vi "Create Contour.vi"(7 "3D Contour Property":T5={"General Property"={"Plot Name"="", "Coordinate System"=enum."Cartesian", "Opacity"=0.0}, "Projection Property"={"Draw XY"=FALSE, "Draw YZ"=FALSE, "Draw XZ"=FALSE}, "Plot Property"={"Line Style"=enum."None", "Line Width"=2.0, "Line Color"=0, "Antialiasing"=FALSE, "Color Ramp Cluster"={"Color Ramp Style"=enum."None", "Color Ramp Array"=[16711934, 393471, 57855, 4390754, 16449346, 16744722, 16711680], "Color Ramp Index"=[45, 91, 133, 175, 219, 255], "Interpolate?"=FALSE, "Logarithm?"=FALSE}}, "Contour Property"={"Contour Type"=enum."Contour", "Axis Basis"=enum."Z-Axis", "Level List"=[], "Level Mode"=enum."Levels", "Levels"=0, "Interval"=0.0}}, 8 "error in (no error)":errorcluster, 9 "Actual Transform In":T1, 10 "Plot Representation In":T3, 11 "Plot Object In":refnum<vi>) -> (0 "error out":errorcluster, 1 "Actual Transform Out":T1, 2 "Plot Representation Out":T3, 3 "Plot Object Out":refnum<vi>, 4 "Contour Object Out":refnum<vi>)   [LabVIEW 2020, in "3D Contour.lvclass"]
uses:
  <vilib>/Math Plots/3D Math Plots/3D Contour/3D Contour/3D Contour.lvclass
  <vilib>/Math Plots/3D Math Plots/3D Contour/3D Contour/Typedef/3D Contour Property.ctl
  <vilib>/Math Plots/3D Math Plots/3D Plot/3D Plot/Typedef/Line Type.ctl
  <vilib>/Math Plots/3D Math Plots/3D Plot/3D Plot/Typedef/Color Ramp Cluster.ctl
  <vilib>/Math Plots/3D Math Plots/3D Plot/3D Plot/Typedef/Plot Representation.ctl
  <vilib>/Math Plots/3D Math Plots/3D Plot/3D Plot/Typedef/Range Clusters.ctl
  <vilib>/Math Plots/3D Math Plots/3D Plot/3D Plot/Typedef/Mesh Data.ctl
  <vilib>/Math Plots/3D Math Plots/3D Plot/3D Plot/Typedef/Actual Transform.ctl
  <vilib>/picture/3D Picture Control/NI_3D Picture Control.lvlib
  <vilib>/Math Plots/3D Math Plots/3D Plot/3D Plot/3D Plot.lvclass
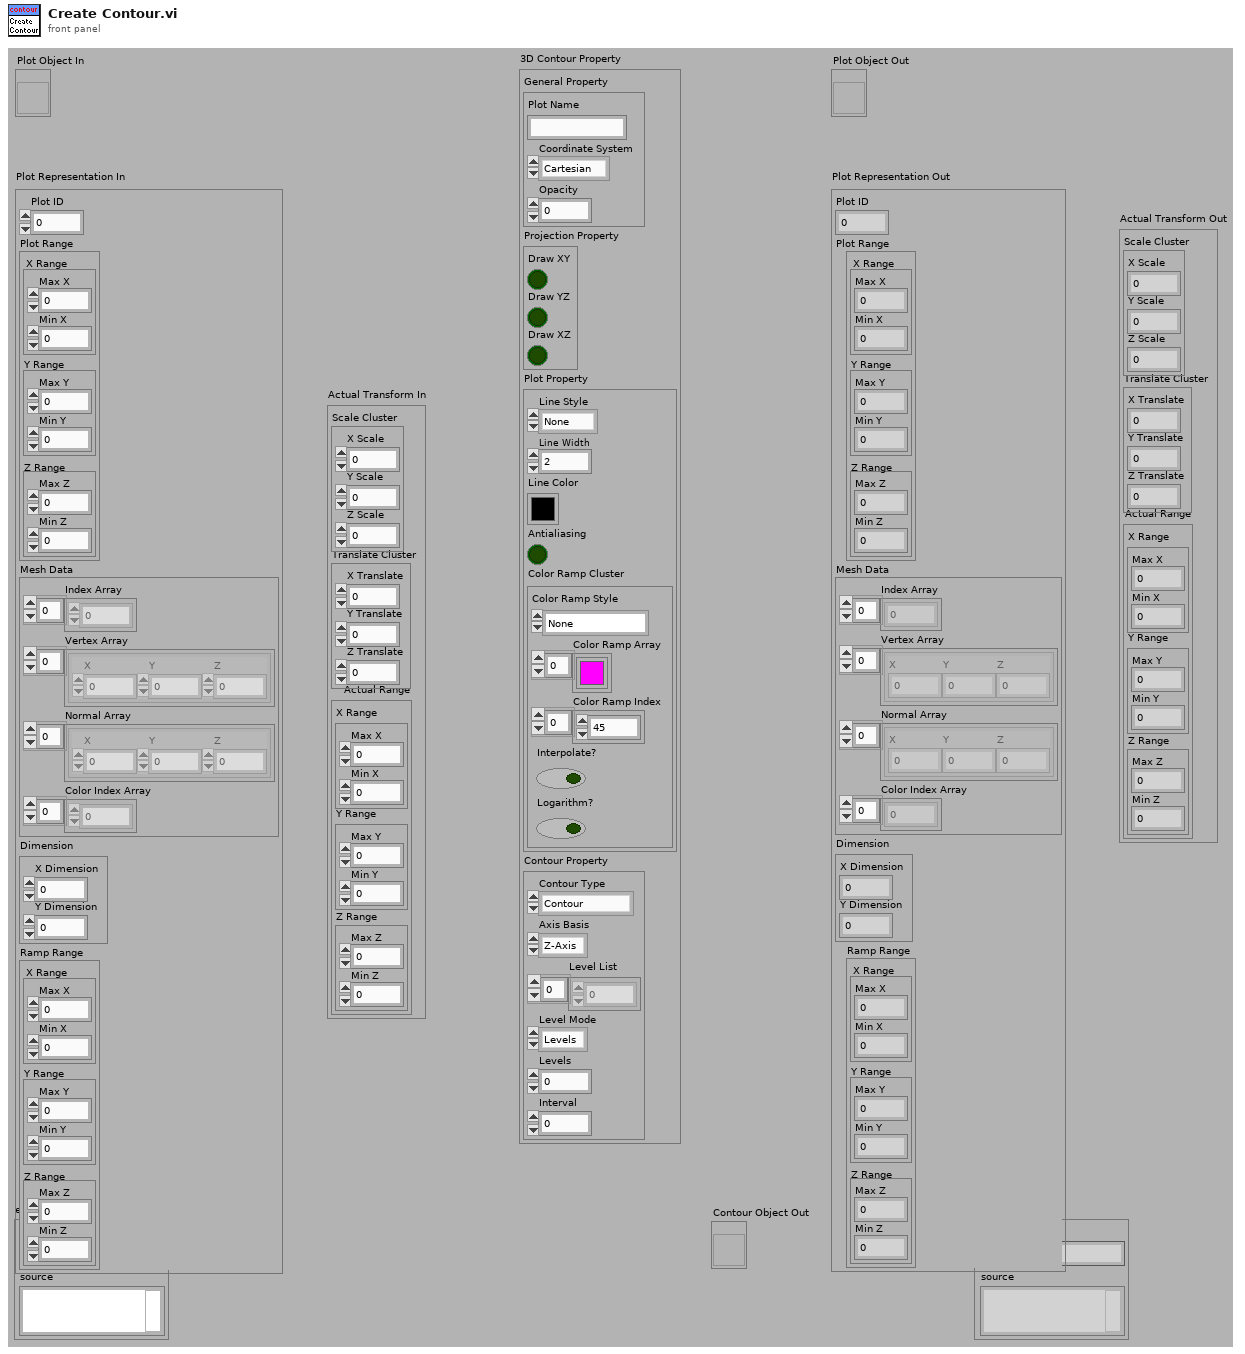
[diagram p1: front panel]
types:
  T1 = typedef "3D Plot.lvclass/Actual Transform.ctl" = cluster{"Scale Cluster":cluster{"X Scale":sgl, "Y Scale":sgl, "Z Scale":sgl}, "Translate Cluster":cluster{"X Translate":sgl, "Y Translate":sgl, "Z Translate":sgl}, "Actual Range":T2}
  T2 = typedef "3D Plot.lvclass/Range Clusters.ctl" = cluster{"X Range":cluster{"Max X":sgl, "Min X":sgl}, "Y Range":cluster{"Max Y":sgl, "Min Y":sgl}, "Z Range":cluster{"Max Z":sgl, "Min Z":sgl}}
  T3 = typedef "3D Plot.lvclass/Plot Representation.ctl" = cluster{"Plot ID":i32, "Plot Range":T2, "Mesh Data":T4, "Dimension":cluster{"X Dimension":i32, "Y Dimension":i32}, "Ramp Range":T2}
  T4 = typedef "3D Plot.lvclass/Mesh Data.ctl" = cluster{"Index Array":u32[], "Vertex Array":cluster{"X":sgl, "Y":sgl, "Z":sgl}[], "Normal Array":cluster{"X":sgl, "Y":sgl, "Z":sgl}[], "Color Index Array":i32[]}
  T5 = typedef "3D Contour.lvclass/3D Contour Property.ctl" = cluster{"General Property":cluster{"Plot Name":string, "Coordinate System":enum16{"Cartesian", "Cylindrical", "Spherical"}, "Opacity":sgl}, "Projection Property":cluster{"Draw XY":bool, "Draw YZ":bool, "Draw XZ":bool}, "Plot Property":cluster{"Line Style":T6, "Line Width":sgl, "Line Color":u32, "Antialiasing":bool, "Color Ramp Cluster":T7}, "Contour Property":cluster{"Contour Type":enum16{"Contour", "Contour with surface"}, "Axis Basis":enum16{"X-Axis", "Y-Axis", "Z-Axis"}, "Level List":sgl[], "Level Mode":enum16{"Levels", "Interval", "Level List"}, "Levels":u16, "Interval":sgl}}
  T6 = typedef "3D Plot.lvclass/Line Type.ctl" = enum16{"None", "Solid", "Dash", "Dot", "Dash Dot"}
  T7 = typedef "3D Plot.lvclass/Color Ramp Cluster.ctl" = cluster{"Color Ramp Style":enum16{"None", "Shaded", "Color spectrum", "Grey scale", "Custom"}, "Color Ramp Array":u32[], "Color Ramp Index":i32[], "Interpolate?":bool, "Logarithm?":bool}
  T8 = enum16{"Points", "Lines", "Line Strip", "Line Loop", "Triangles", "Triangle Strip", "Triangle Fan", "Quads", "Quad Strip", "Polygon"}
  T9 = cluster{"Contour Type":enum16{"Contour", "Contour with surface"}, "Axis Basis":enum16{"X-Axis", "Y-Axis", "Z-Axis"}, "Level List":sgl[], "Level Mode":enum16{"Levels", "Interval", "Level List"}, "Levels":u16, "Interval":sgl}
  T10 = enum16{"Overall", "Per Primitive", "Per Vertex", "Binding Off"}
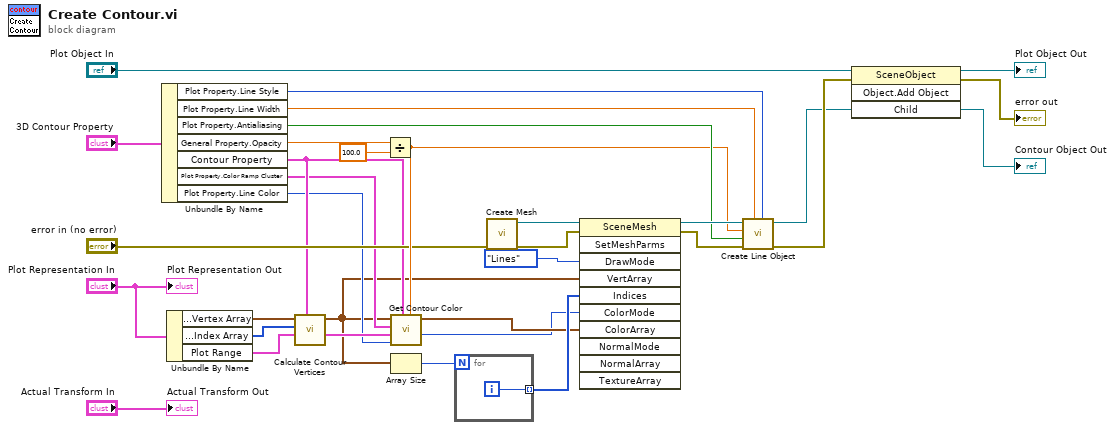
[diagram p0: block diagram]
diagram:
  n1 = Unbundle By Name("3D Contour Property") -> ("Plot Property.Line Style"=w13:T6, "Plot Property.Line Width"=w14:sgl, "Plot Property.Antialiasing"=w12:bool, "General Property.Opacity"=w20:sgl, "Contour Property"=w4:T9, "Plot Property.Color Ramp Cluster"=w3:T7, "Plot Property.Line Color"=w2:u32)
  n2 = Unbundle By Name("Plot Representation In") -> ("Mesh Data.Vertex Array"=w8:cluster{"X":sgl, "Y":sgl, "Z":sgl}[], "Mesh Data.Index Array"=w7:u32[], "Plot Range"=w6:T2)
  n3 = call <vilib>:"Calculate Contour Vertices.vi"("Contour Property In"=w4, "Range In"=w6, "Mesh Index Array"=w7, "Mesh Vertex Array In"=w8) -> ("Range Out"=w5:T2, "Contour Vertex Array Out"=w1:cluster{"X":sgl, "Y":sgl, "Z":sgl}[])  [unwired: 1 in, 5 out]
  n4 = Divide(x=w20, y=sgl 100.0) -> (x/y=w11:sgl)
  n5 = call <vilib>:"Get Contour Color.vi"("Opacity"=w11, "Contour Property In"=w4, "Line Color"=w2, "Actual Range"=w5, "Color Ramp Cluster"=w3, "Contour Vertex Array"=w1) -> ("Color Binding Mode"=w22:T10, "Color Array Out"=w23:cluster{"R":sgl, "G":sgl, "B":sgl, "A":sgl}[])  [unwired: 4 out]
  n6 = Array Size(array=w1) -> (size(s)=w26:i32)
  n7 = for {
    N: w26 -> [_]
    tunnel: [w34] -> w24 mode=indexing
    i -> [w34]
  }
  n8 = call <vilib>:"Create Mesh.vi"("error in (no error)"="error in (no error)") -> ("error out"=w25:errorcluster, "New Mesh Refnum"=w28:refnum<vi>)  [unwired: 9 out]
  n9 = invoke class="SceneMesh" method="SetMeshParms"(reference=w28, error in=w25, "DrawMode"=T8."Lines" ("Draw Mode"), "VertArray"=w1, "Indices"=w24, "ColorMode"=w22, "ColorArray"=w23) -> (reference out=w18:refnum<vi>, error out=w17:errorcluster)  [unwired: 4 in, 9 out]
  n10 = call <vilib>:"Create Line Object.vi"("Line Style"=w13, "Line Width"=w14, "error in (no error)"=w17, "Antialiasing"=w12, "Alpha"=w11, "Mesh Ref In"=w18) -> ("error out"=w16:errorcluster, "Object Ref Out"=w15:refnum<vi>)  [unwired: 4 out]
  n11 = invoke class="SceneObject" method="Object.Add Object"(reference="Plot Object In", error in=w16, "Child"=w15) -> (reference out=→"Plot Object Out":refnum<vi>, error out=→"error out":errorcluster, "Child"=→"Contour Object Out":refnum<vi>)  [unwired: 1 in, 1 out]
  "Plot Representation Out" <- "Plot Representation In"
  "Actual Transform Out" <- "Actual Transform In"
